vi "UI.UpdateWaveform.vi"(8 "error in (no error)":errorcluster, 11 "State Variables":T1={"Aliases.All"=[], "Aliases.Outputs"=[], "UI.Sequence#ofColumns"=0, "SysDef.Path"=path "", "UI.SequenceRef"=refnum, "UI.StepInformationRef"=refnum, "UI.AbortRef"=refnum, "UI.GraphRef"=refnum, "UI.ViewRef"=refnum, "UI.IterationsRef"=refnum, "UI.IterationInformationRef"=refnum, "INI.Settings"={"Build Location"=path "C:/Simple Sequence Editor/SequenceRepo", "LoggingLocation"=path ""}}) -> (0 "error out":errorcluster, 2 "Wavefrom":waveform(dbl)[](array[waveform]), 3 "State Variables out":T1={"Aliases.All"=[], "Aliases.Outputs"=[], "UI.Sequence#ofColumns"=0, "SysDef.Path"=path "", "UI.SequenceRef"=refnum, "UI.StepInformationRef"=refnum, "UI.AbortRef"=refnum, "UI.GraphRef"=refnum, "UI.ViewRef"=refnum, "UI.IterationsRef"=refnum, "UI.IterationInformationRef"=refnum, "INI.Settings"={"Build Location"=path "C:/Simple Sequence Editor/SequenceRepo", "LoggingLocation"=path ""}})   [LabVIEW 2013, in "Simple Sequence Editor.lvlib"]
uses:
  Simple Sequence Editor.lvlib
  Types/StateVariables.ctl
  Types/ChannelProperties.ctl
  Types/INI.Settings
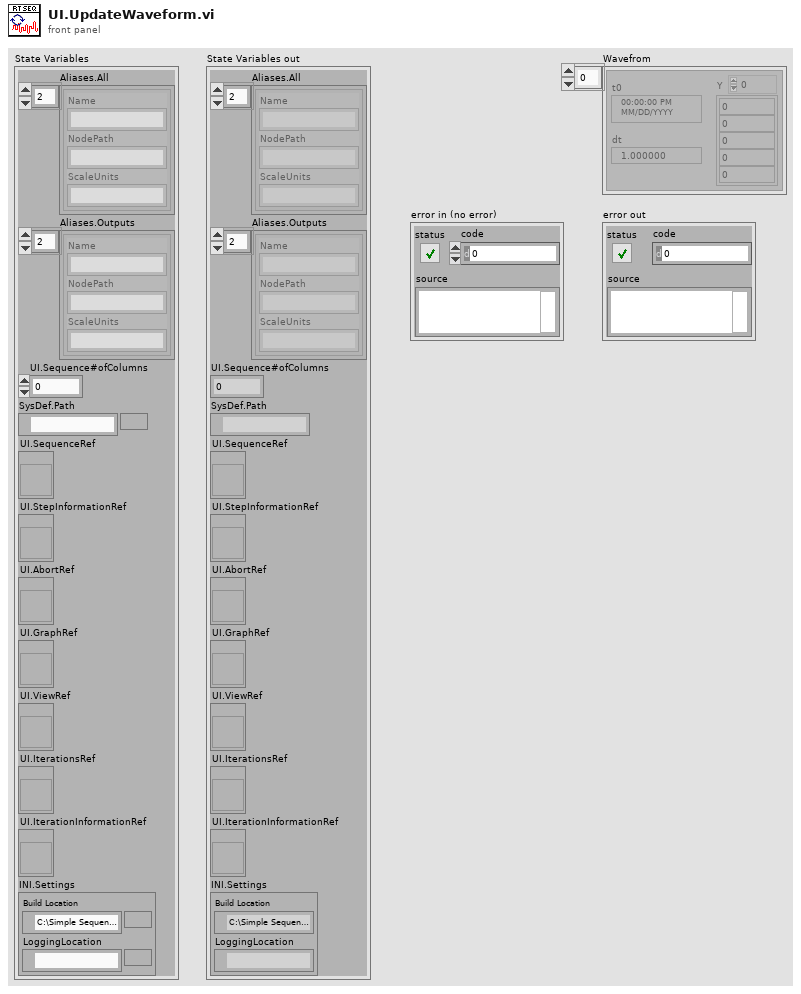
[diagram p1: front panel]
types:
  T1 = typedef "Simple Sequence Editor.lvlib/StateVariables.ctl" = cluster{"Aliases.All":T2[], "Aliases.Outputs":T2[], "UI.Sequence#ofColumns":i32, "SysDef.Path":path, "UI.SequenceRef":refnum<vi>, "UI.StepInformationRef":refnum<vi>, "UI.AbortRef":refnum<vi>, "UI.GraphRef":refnum<vi>, "UI.ViewRef":refnum<vi>, "UI.IterationsRef":refnum<vi>, "UI.IterationInformationRef":refnum<vi>, "INI.Settings":T3}
  T2 = typedef "Simple Sequence Editor.lvlib/ChannelProperties.ctl" = cluster{"Name":string, "NodePath":string, "ScaleUnits":string}
  T3 = typedef "Simple Sequence Editor.lvlib/INI.Settings" = cluster{"Build Location":path, "LoggingLocation":path}
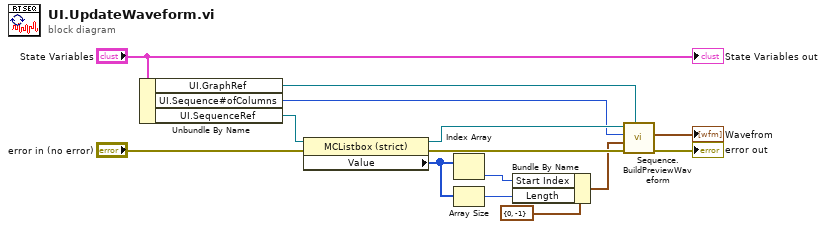
[diagram p0: block diagram]
diagram:
  n1 = Unbundle By Name("State Variables") -> ("UI.GraphRef"=w14:refnum<vi>, "UI.Sequence#ofColumns"=w1:i32, "UI.SequenceRef"=w7:refnum<vi>)
  n2 = property class="MCListbox (strict)"(reference=w7, error in="error in (no error)") -> (reference out=w2:refnum<vi>, error out=w9:errorcluster, "Value"=w12:i32[])
  n3 = Index Array(array=w12) -> (element=w13:i32)  [unwired: 1 in]
  n4 = Array Size(array=w12) -> (size(s)=w11:i32)
  n5 = Bundle By Name(cluster=cluster{"Start Index":i32, "Length":i32} {"Start Index"=0, "Length"=-1} ("Rows"), "Start Index"=w13, "Length"=w11) -> (w4:cluster{"Start Index":i32, "Length":i32})
  n6 = call "Sequence.BuildPreviewWaveform.vi"("WaveformGraph in"=w14, "error in (no error)"=w9, "Rows"=w4, "UI.Sequence#ofColumns"=w1, "SequenceRef"=w2) -> ("error out"=→"error out":errorcluster, "Wavefrom"=→"Wavefrom":waveform(dbl)[])  [unwired: 5 in]
  "State Variables out" <- "State Variables"
